vi "Advance Query Adjust In built table.vi"(8 "error in (no error)":errorcluster, 10 "Database in":refnum<class "Database.lvclass">, 11 "RequestRestUI":refnum<class "RequestRestUI.lvclass">) -> (0 "error out":errorcluster, 3 "RequestRestUI out":refnum<class "RequestRestUI.lvclass">)   [LabVIEW 2015, in "RequestRestUI.lvclass"]
uses:
  RequestRestUI.lvclass
  DatabaseManagement/Database.lvclass
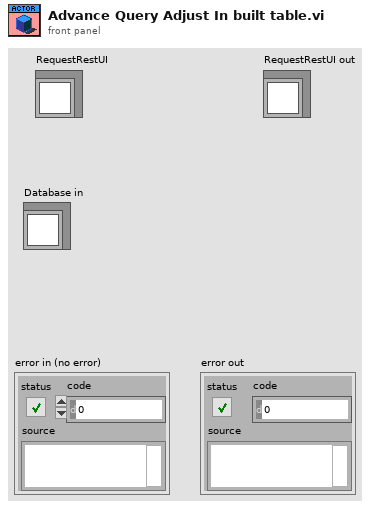
[diagram p1: front panel]
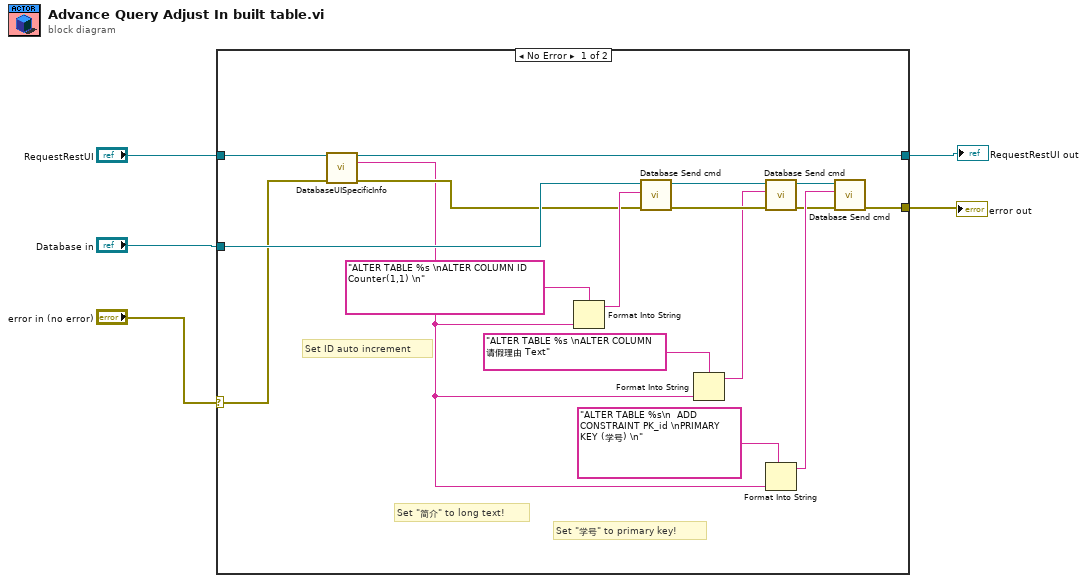
[diagram p0: block diagram]
diagram:
  n1 = case shown="No Error" "error in (no error)" {
    selector: "error in (no error)" -> [w10 w24]
    tunnel: [w22 w24] -> w1
    tunnel: "RequestRestUI" -> [w12 w23]
    tunnel: "Database in" -> [w11 _]
    tunnel: [w7 w23] -> w2
    frame No Error {
      # "Set \"学号\" to primary key!"
      # "Set \"简介\" to long text!"
      # "Set ID auto increment"
      n2 = call-dynamic "DatabaseUISpecificInfo.vi"("requestActor in"=w12, "error in (no error)"=w10) -> ("requestActor out"=w7:refnum<class "RequestRestUI.lvclass">, "TableName"=w8:string, "error out"=w9:errorcluster)  [unwired: 9 in, 2 out]
      n3 = Format Into String(format string="ALTER TABLE %s \nALTER COLUMN ID Counter(1,1) \n" ("SQL query"), w8) -> (resulting string=w18:string)  [unwired: 2 in, 1 out]
      n4 = call "Database Send cmd.vi"("error in (no error)"=w9, "SQL query"=w18, "Database in"=w11) -> ("error out"=w15:errorcluster, "Database out"=w16:refnum<class "Database.lvclass">)  [unwired: 7 in]
      n5 = Format Into String(format string="ALTER TABLE %s \nALTER COLUMN 请假理由 Text" ("SQL query"), w8) -> (resulting string=w6:string)  [unwired: 2 in, 1 out]
      n6 = call "Database Send cmd.vi"("error in (no error)"=w15, "SQL query"=w6, "Database in"=w16) -> ("error out"=w13:errorcluster, "Database out"=w14:refnum<class "Database.lvclass">)  [unwired: 7 in]
      n7 = Format Into String(format string="ALTER TABLE %s\n  ADD CONSTRAINT PK_id \nPRIMARY KEY (学号) \n" ("SQL query"), w8) -> (resulting string=w17:string)  [unwired: 2 in, 1 out]
      n8 = call "Database Send cmd.vi"("error in (no error)"=w13, "SQL query"=w17, "Database in"=w14) -> ("error out"=w22:errorcluster)  [unwired: 7 in, 1 out]
    }
    frame Error {
    }
  }
  "error out" <- w1
  "RequestRestUI out" <- w2
